vi "Settings Dialog.vi"(8 "error in (no error)":errorcluster, 11 "Configuration in":T1={"Hardware Configuration"={"Physical Channel"="", "Maximum Input"=0.0, "Minimum Input"=0.0, "Sample Rate"=0.0, "Number of Samples"=0}, "Analysis Configuration"={"Statistics"=TRUE}, "New Data Behavior"=enum."Replace"}) -> (0 "error out":errorcluster, 2 "UI Refresh Needed?":bool, 3 "Configuration out":T1={"Hardware Configuration"={"Physical Channel"="", "Maximum Input"=0.0, "Minimum Input"=0.0, "Sample Rate"=0.0, "Number of Samples"=0}, "Analysis Configuration"={"Statistics"=TRUE}, "New Data Behavior"=enum."Replace"})   [LabVIEW 2018]
doc: "Dialog for selecting user specified settings."
uses:
  controls/User Specified Data.ctl
  controls/HW Configuration.ctl
  controls/Analysis Configuration.ctl
  controls/New Data Behavior.ctl
panel:
  in  "Number of Samples":i32=1000
  in  "Sample Rate":dbl=10000.0
  in  "Minimum Input":dbl=-10.0
  in  "Maximum Input":dbl=10.0
  in  "Physical Channel":tag="Dev1/ai0"
  in  "New Data Behavior":u16(ring) items=["Replace", "Overlay", "Append"]
  in  "Cancel Button":bool
  in  "OK Button":bool
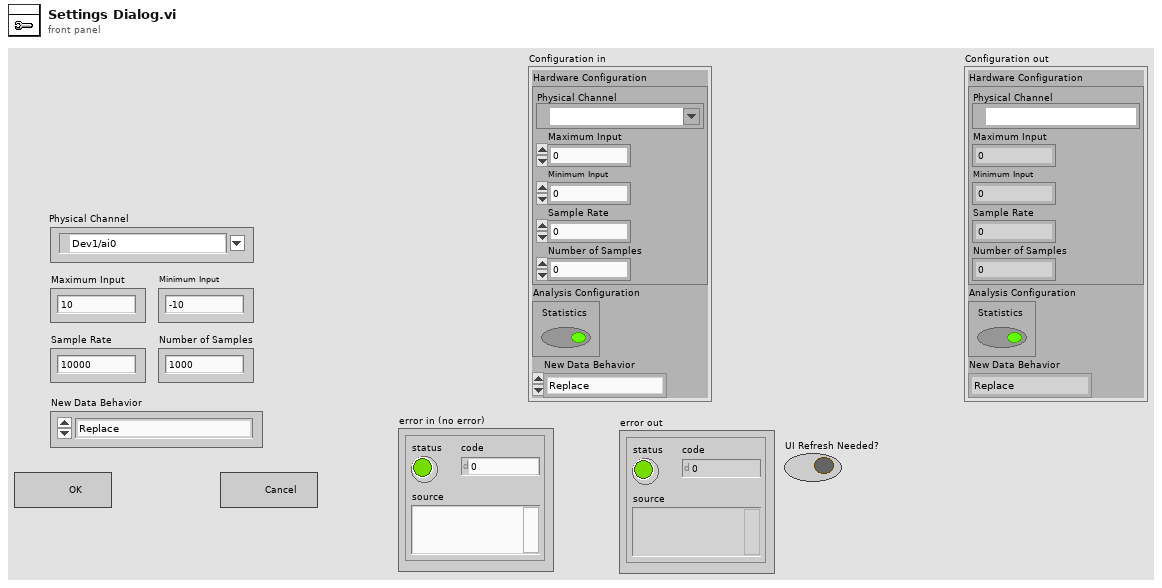
[diagram p1: front panel]
types:
  T1 = typedef "User Specified Data.ctl" = cluster{"Hardware Configuration":T2, "Analysis Configuration":T3, "New Data Behavior":T4}
  T2 = typedef "HW Configuration.ctl" = cluster{"Physical Channel":tag, "Maximum Input":dbl, "Minimum Input":dbl, "Sample Rate":dbl, "Number of Samples":i32}
  T3 = typedef "Analysis Configuration.ctl" = cluster{"Statistics":bool}
  T4 = typedef "New Data Behavior.ctl" = enum16{"Replace", "Overlay", "Append"}
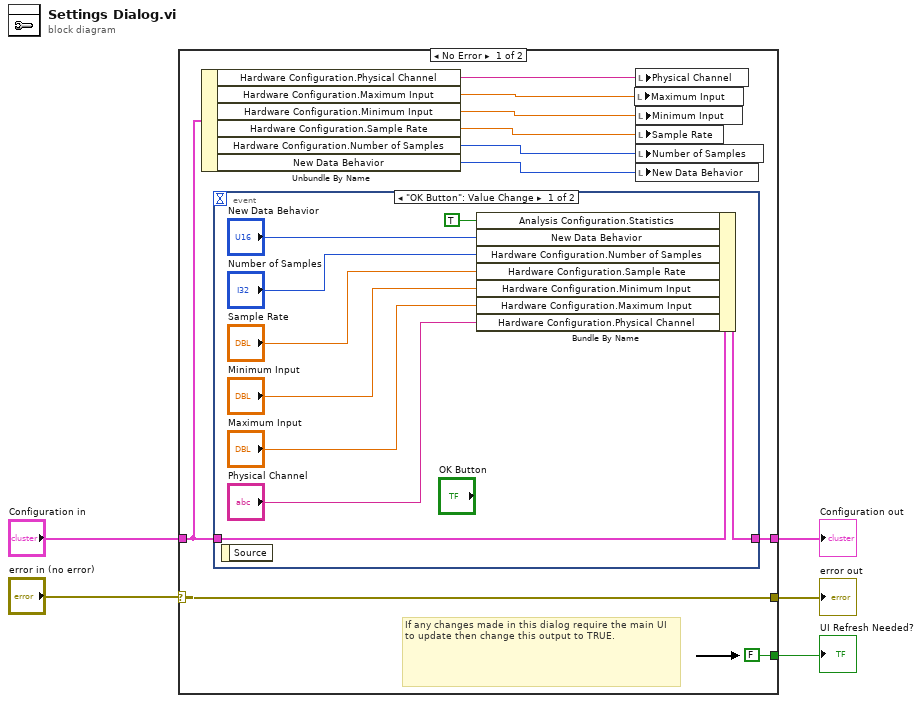
[diagram p0: block diagram]
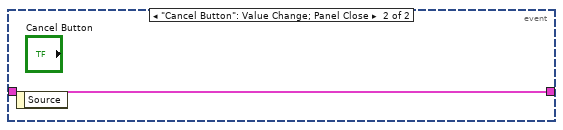
[diagram p2: hidden frame]
diagram:
  n1 = case shown="No Error" "error in (no error)" {
    selector: "error in (no error)" -> [w13 w27]
    tunnel: [w13 w27] -> w4
    tunnel: "Configuration in" -> [w12 w26]
    tunnel: [w15 w26] -> w2
    tunnel: [FALSE ("UI Refresh Needed?") _] -> w1
    frame No Error {
      # "If any changes made in this dialog require the main UI to update then change this output to TRUE."
      n2 = Unbundle By Name(w12) -> ("Hardware Configuration.Physical Channel"=w11:tag, "Hardware Configuration.Maximum Input"=w10:dbl, "Hardware Configuration.Minimum Input"=w9:dbl, "Hardware Configuration.Sample Rate"=w8:dbl, "Hardware Configuration.Number of Samples"=w7:i32, "New Data Behavior"=w6:T4)
      n3 = event shown="[0] \"OK Button\": Value Change" {
        selector: _ -> [_ _]
        dyn-events: _ -> [_ _]
        timeout: _ -> [_ _]
        tunnel: [w24 w25] -> w15
        tunnel: w12 -> [w22 w25]
        event "OK Button": Value Change {
          n4 = event-data() -> ()  [unwired: 1 in, 1 out]
          n5 = Bundle By Name(cluster=w22, "Analysis Configuration.Statistics"=TRUE, "New Data Behavior"="New Data Behavior", "Hardware Configuration.Number of Samples"="Number of Samples", "Hardware Configuration.Sample Rate"="Sample Rate", "Hardware Configuration.Minimum Input"="Minimum Input", "Hardware Configuration.Maximum Input"="Maximum Input", "Hardware Configuration.Physical Channel"="Physical Channel") -> (w24:T1)
        }
        event "Cancel Button": Value Change; Panel Close {
          n6 = event-data() -> ()  [unwired: 1 in, 1 out]
        }
      }
      n7 = local write "Maximum Input"(w10) -> ()
      n8 = local write "Physical Channel"(w11) -> ()
      n9 = local write "Minimum Input"(w9) -> ()
      n10 = local write "Sample Rate"(w8) -> ()
      n11 = local write "Number of Samples"(w7) -> ()
      n12 = local write "New Data Behavior"(w6) -> ()
    }
    frame Error {
    }
  }
  "UI Refresh Needed?" <- w1
  "error out" <- w4
  "Configuration out" <- w2
